vi "OA Get Float.vi"(9 "fFloatValue":sgl, 10 "pcModeParam":string, 11 "pcModeName":string) -> (1 "fFloatValue out":sgl, 3 "function return":u32)   [LabVIEW 2018, in "Copy of Andor SDK.lvlib"]
doc: "EXPNETTYPE unsigned int WINAPI OA_GetFloat(const char * const pcModeName, const char * const pcModeParam, float * fFloatValue);"
uses:
  Copy of Andor SDK.lvlib
  <userlib>/Andor SDK/ATMCD32D.dll
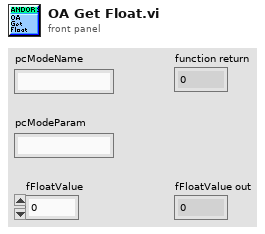
[diagram p1: front panel]
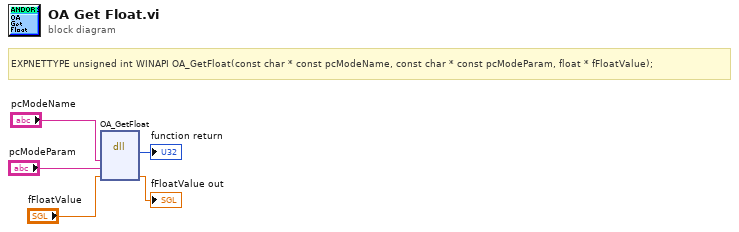
[diagram p0: block diagram]
diagram:
  # "EXPNETTYPE unsigned int WINAPI OA_GetFloat(const char * const pcModeName, const char * const pcModeParam, float * fFloatValue);"
  n1 = dll-call lib="C:/Program Files (x86)/National Instruments/LabVIEW 2018/user.lib/Andor SDK/ATMCD32D.*" fn="OA_GetFloat"("pcModeName"="pcModeName", "pcModeParam"="pcModeParam", "fFloatValue"="fFloatValue") -> (→"function return":u32, "fFloatValue"=→"fFloatValue out":sgl)  [unwired: 5 in, 2 out]
